vi "太阳能控制器界面.vi"() -> ()   [LabVIEW 2016, in "环境动力监测库.lvlib"]
uses:
  <vilib>/Utility/miscctls.llb/LVPointTypeDef.ctl
  <vilib>/Utility/config.llb/NI_LVConfig.lvlib
  <vilib>/ptbypt/NI_PtbyPt.lvlib
panel:
  in  "报警设置":bool
  in  "MPPT-24 串口":refnum<visa-resource-name> caption="MPPT-24"
  in  "MPPT-12 串口":refnum<visa-resource-name> caption="MPPT-12"
  out "充放电信息 2":T1 caption="充放电信息_KWH" {"总累计充电量" format="%.2f"; "当年累计充电量" format="%.2f"; "当月累计充电量" format="%.2f"; "当日累计充电量" format="%.2f"; "当年累计用电量" format="%.2f"; "当月累计用电量" format="%.2f"; "当日累计用电量" format="%.2f"}
  out "状态 2":string caption="状态"
  out "状态":string
  out "充放电信息":T1 caption="充放电信息_KWH" {"总累计充电量" format="%.2f"; "当年累计充电量" format="%.2f"; "当月累计充电量" format="%.2f"; "当日累计充电量" format="%.2f"; "当年累计用电量" format="%.2f"; "当月累计用电量" format="%.2f"; "当日累计用电量" format="%.2f"}
  out "通讯状态 3":bool
  out "通讯状态 2":bool
  out "控制器信息 2":cluster{"设备温度℃":dbl} caption="控制器信息"
  out "直流负载信息 2":cluster{"负载电压V":dbl, "负载电流A":dbl, "负载功率W":dbl} caption="直流负载信息"
  out "蓄电池信息 2":T2 caption="蓄电池信息"
  out "阵列信息 2":cluster{"阵列电压V":dbl, "阵列电流A":dbl, "发电功率W":dbl} caption="阵列信息"
  out "控制器信息":cluster{"设备温度℃":dbl}
  out "直流负载信息":cluster{"负载电压V":dbl, "负载电流A":dbl, "负载功率W":dbl}
  out "蓄电池信息":T2
  out "阵列信息":cluster{"阵列电压V":dbl, "阵列电流A":dbl, "发电功率W":dbl}
  # "MPPT-12"
  # "MPPT-24"
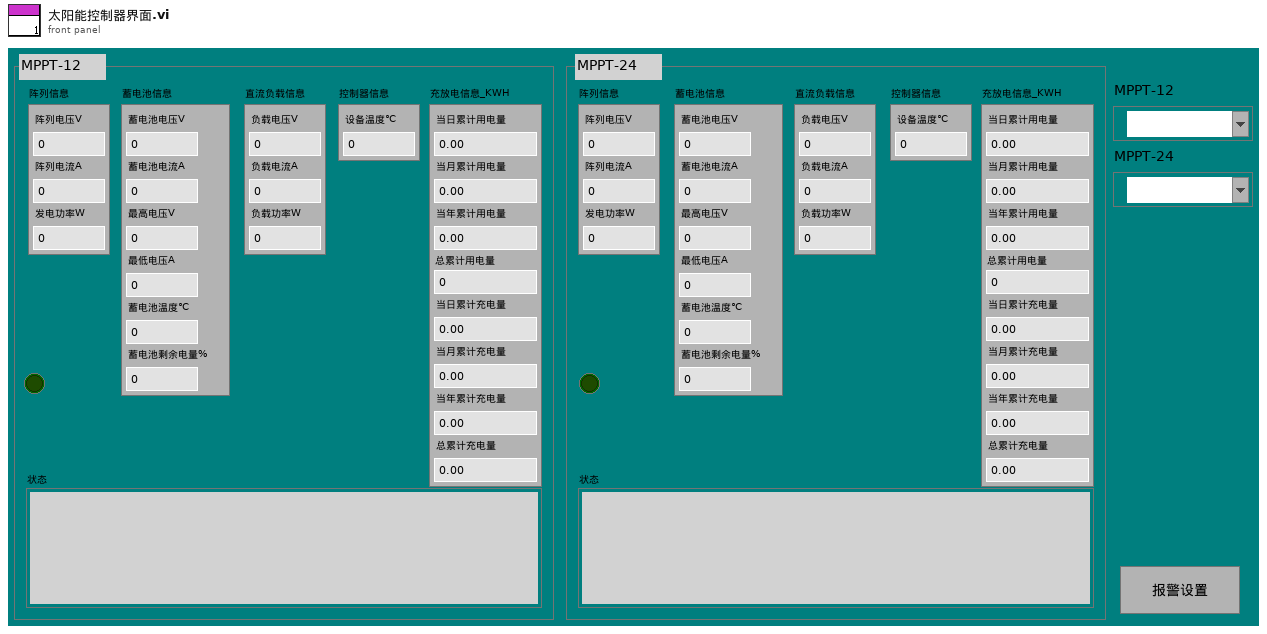
[diagram p1: front panel]
types:
  T1 = cluster{"当日累计用电量":sgl, "当月累计用电量":sgl, "当年累计用电量":sgl, "总累计用电量":sgl, "当日累计充电量":sgl, "当月累计充电量":sgl, "当年累计充电量":sgl, "总累计充电量":sgl}
  T2 = cluster{"蓄电池电压V":dbl, "蓄电池电流A":dbl, "最高电压V":dbl, "最低电压A":dbl, "蓄电池温度℃":dbl, "蓄电池剩余电量%":dbl}
  T3 = typedef "LVPointTypeDef.ctl" = cluster{"Horizontal":i16, "Vertical":i16}
  T4 = typedef "NI_LVConfig.lvlib/Config Data RefNum.ctl" = refnum<k1>
  T5 = enum8{"Enabled", "Disabled", "Disabled and Grayed Out"}
  T6 = cluster{"蓄电池状态":string, "阵列状态":string, "充电状态":string, "负载状态":string, "设备状态":string}
  T7 = cluster{"状态":cluster{"蓄电池状态":string, "阵列状态":string, "充电状态":string, "负载状态":string, "设备状态":string}, "充放电信息":cluster{"当日累计用电量":sgl, "当月累计用电量":sgl, "当年累计用电量":sgl, "总累计用电量":sgl, "当日累计充电量":sgl, "当月累计充电量":sgl, "当年累计充电量":sgl, "总累计充电量":sgl}, "控制器信息":cluster{"设备温度℃":dbl}, "蓄电池信息":cluster{"蓄电池电压V":dbl, "蓄电池电流A":dbl, "最高电压V":dbl, "最低电压A":dbl, "蓄电池温度℃":dbl, "蓄电池剩余电量%":dbl}, "阵列信息":cluster{"阵列电压V":dbl, "阵列电流A":dbl, "发电功率W":dbl}, "直流负载信息":cluster{"负载电压V":dbl, "负载电流A":dbl, "负载功率W":dbl}, "error out":errorcluster}
  T8 = cluster{"时间":timestamp, "阵列电压_V":dbl, "阵列电流_A":dbl, "发电功率_W":dbl, "蓄电池电压_V":dbl, "蓄电池电流_A":dbl, "最高电压_V":dbl, "最低电压_A":dbl, "蓄电池温度_℃":dbl, "蓄电池剩余电量_%":dbl, "负载电压_V":dbl, "负载电流_A":dbl, "负载功率_W":dbl, "设备温度_℃":dbl, "当日累计用电量_KWH":dbl, "当月累计用电量_KWH":dbl, "当年累计用电量_KWH":dbl, "总累计用电量_KWH":dbl, "当日累计充电量_KWH":dbl, "当月累计充电量_KWH":dbl, "当年累计充电量_KWH":dbl, "总累计充电量_KWH":dbl}
  T9 = typedef "LVDateTimeRec.ctl" = cluster{"秒数的小数部分":dbl, "秒":i32, "分":i32, "时":i32, "日":i32, "月":i32, "年":i32, "天数（周）":i32, "天数（年）":i32, "DST":i32}
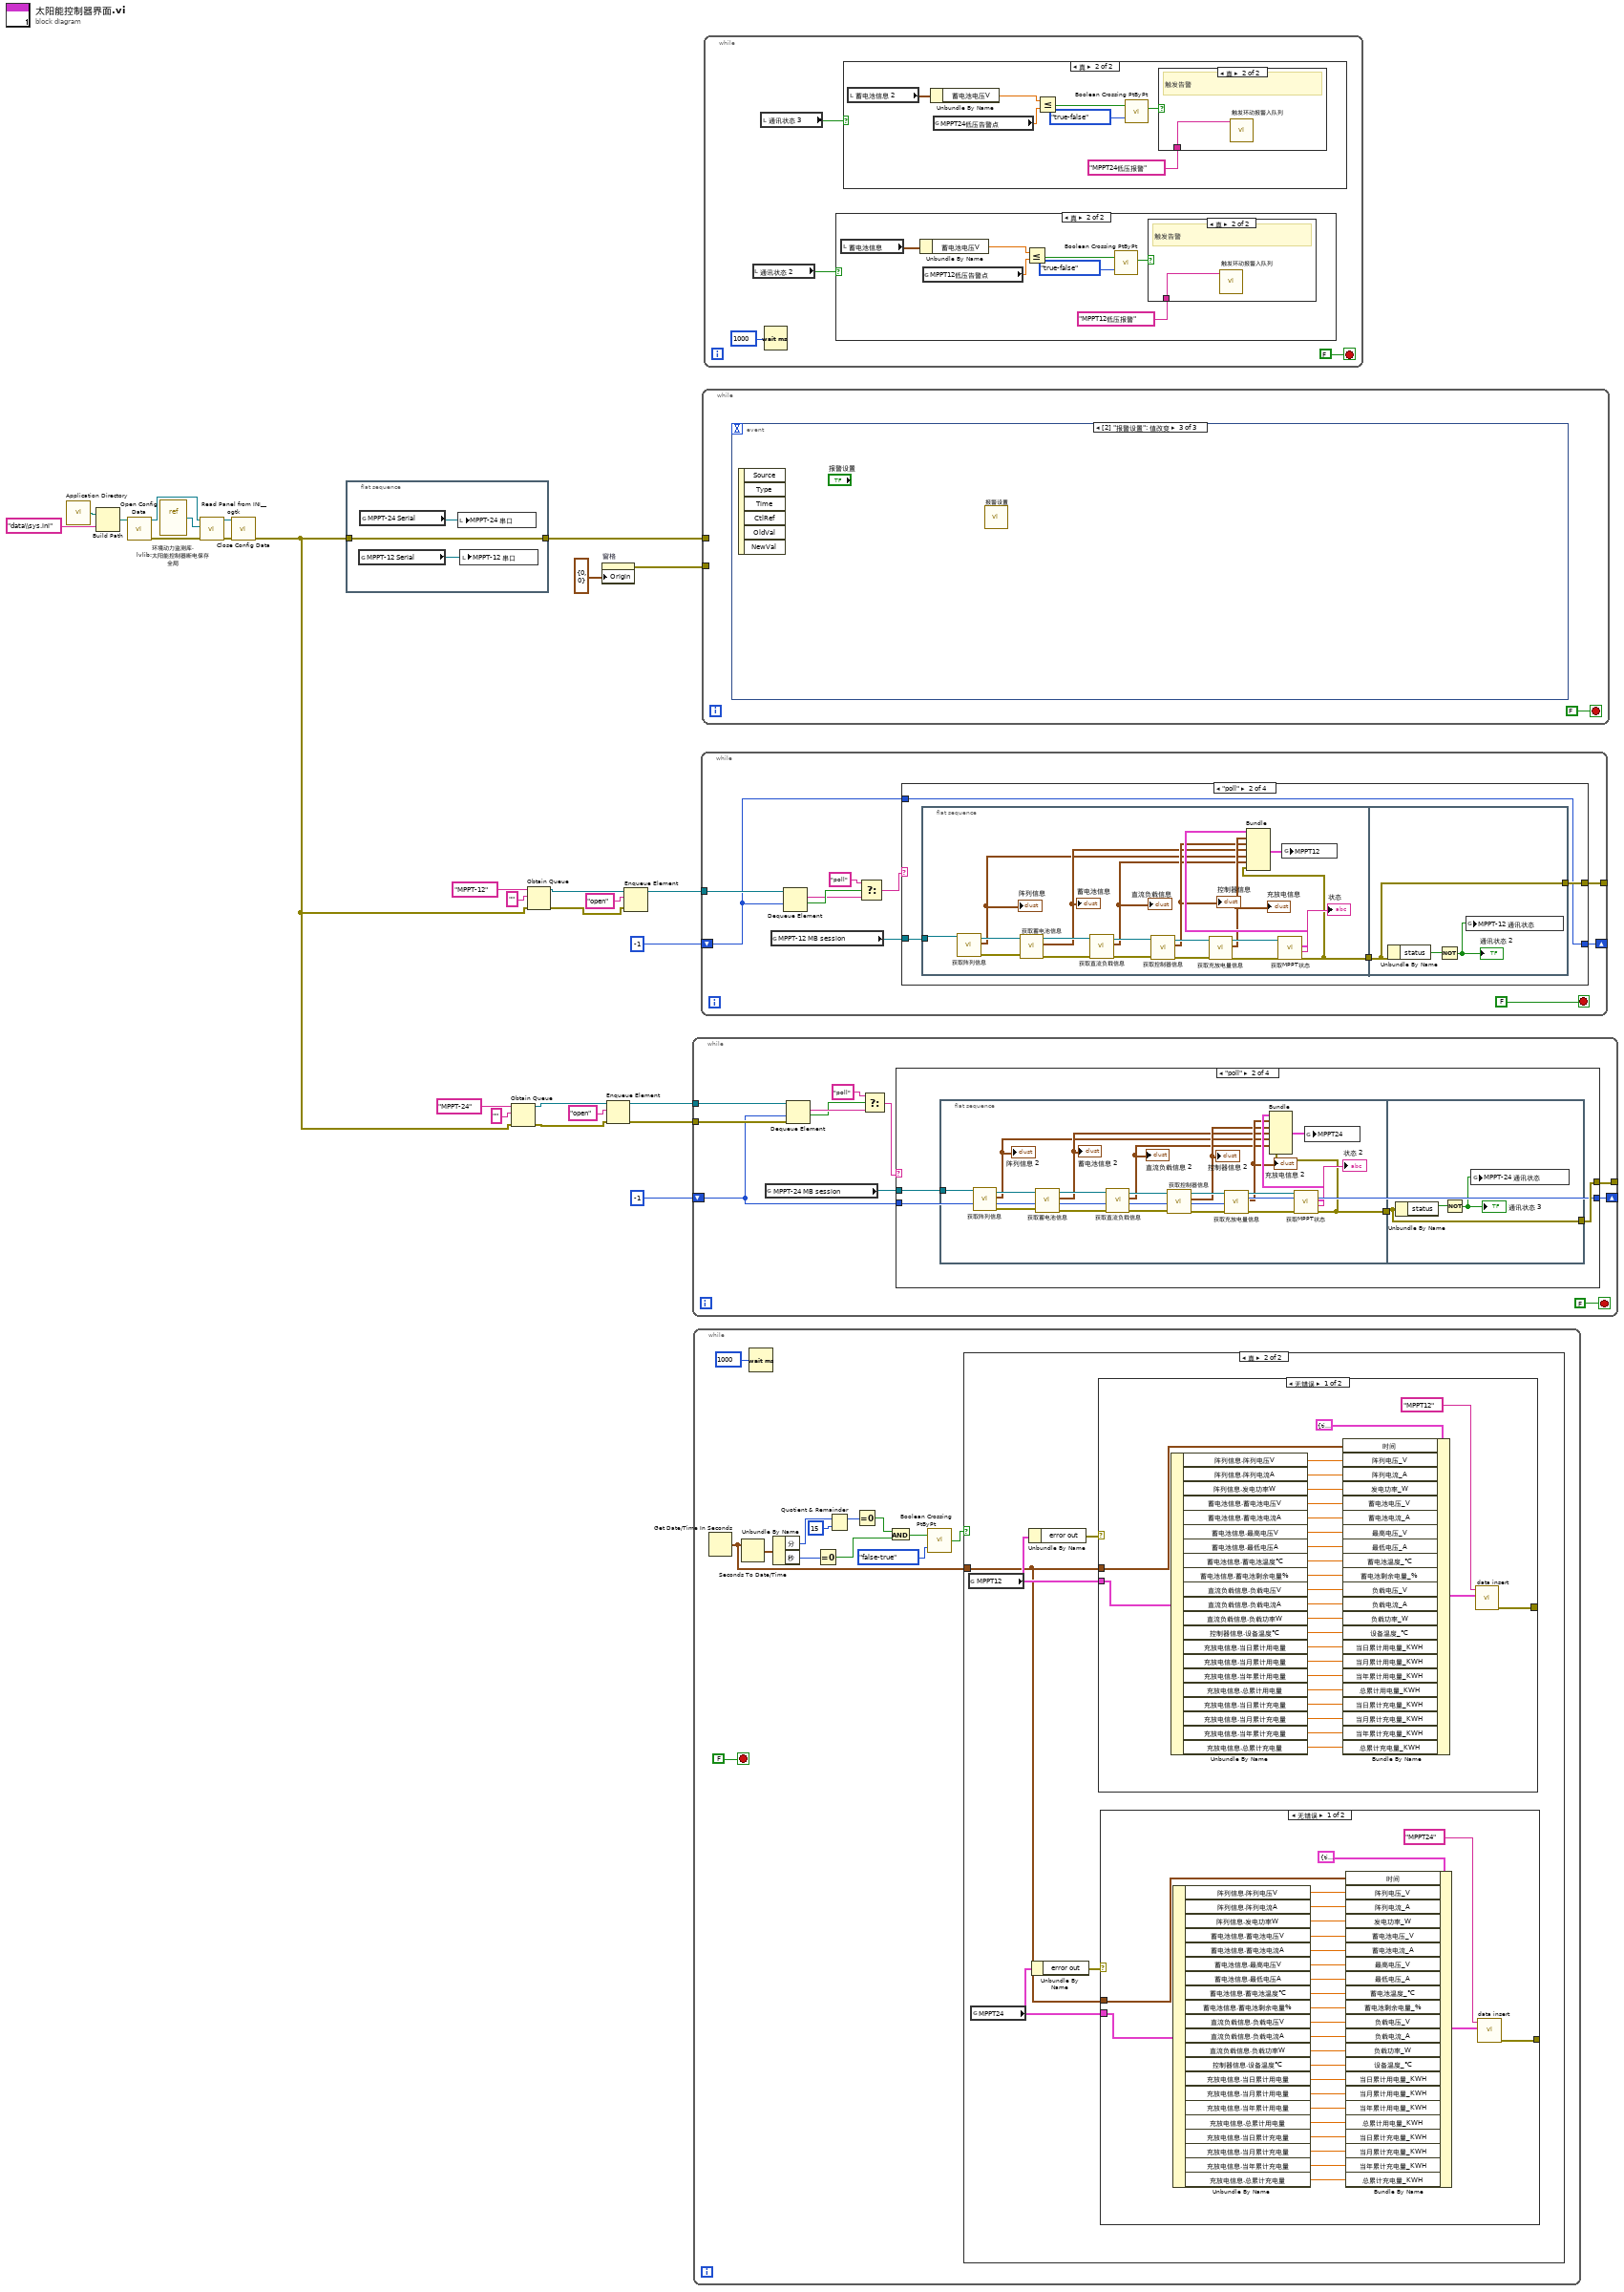
[diagram p0: block diagram]
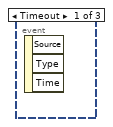
[diagram p9: hidden frame]
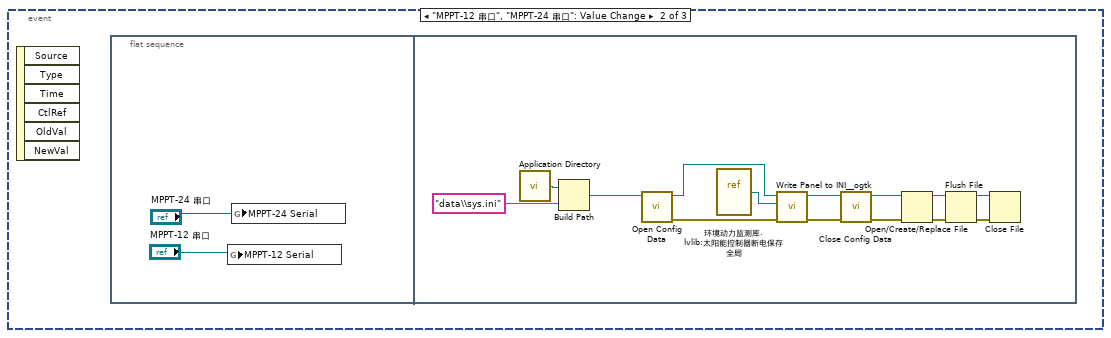
[diagram p10: hidden frame]
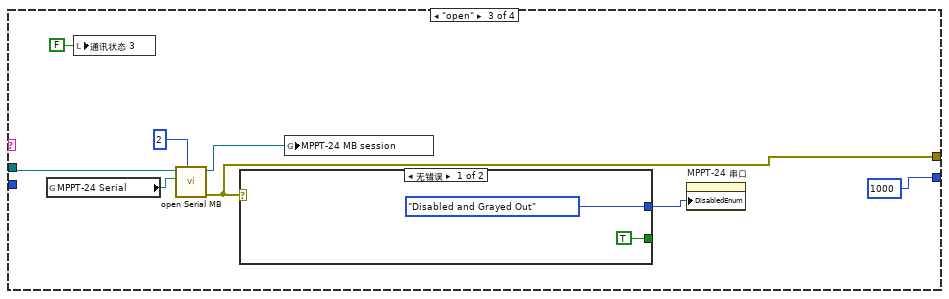
[diagram p12: hidden frame]
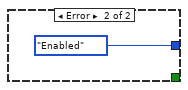
[diagram p13: hidden frame]
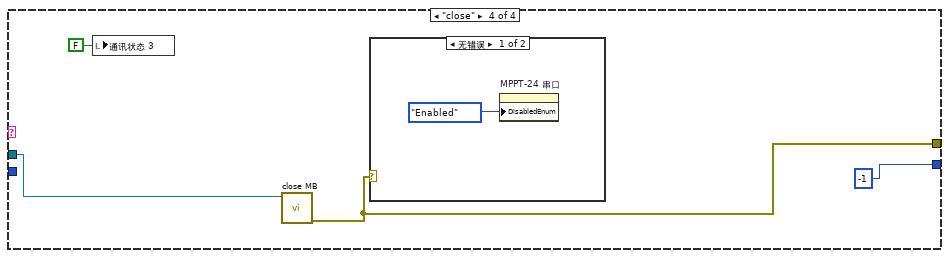
[diagram p14: hidden frame]
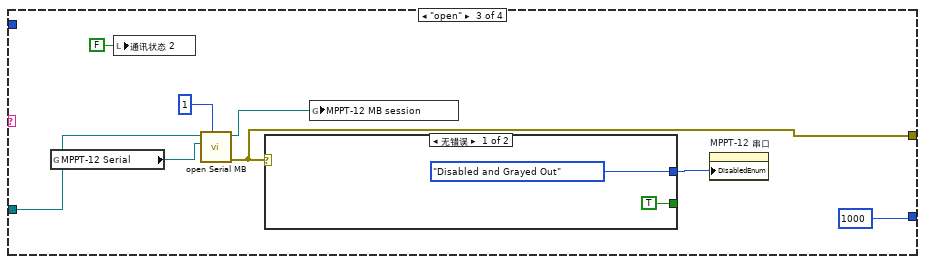
[diagram p17: hidden frame]
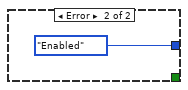
[diagram p18: hidden frame]
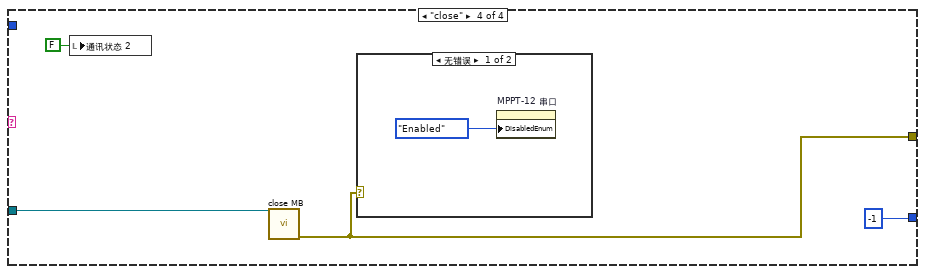
[diagram p19: hidden frame]
diagram:
  n1 = call <vilib>:"Application Directory.vi"() -> ("Application Directory"=w16:path)
  n2 = Build Path(base path=w16, name or relative path="data\\sys.ini" ("名称或相对路径")) -> (appended path=w18:path)
  n3 = call <vilib>:"Open Config Data.vi"("configuration file path"=w18) -> ("error out"=w22:errorcluster, "refnum"=w19:T4)  [unwired: 8 in, 1 out]
  n4 = vi-ref "环境动力监测库.lvlib:太阳能控制器断电保存全局.vi"() -> (w20:refnum<vi>)
  n5 = call <userlib>:"Read Panel from INI__ogtk.vi"("error in (no error)"=w22, "VI ref"=w20, "refnum"=w19) -> ("error out"=w15:errorcluster, "refnum out"=w21:T4)  [unwired: 7 in]
  n6 = call <vilib>:"Close Config Data.vi"("error in (no error)"=w15, "refnum"=w21) -> ("error out"=w2:errorcluster)  [unwired: 8 in, 1 out]
  n7 = flat-sequence {
    tunnel: w2 -> [w28]
    tunnel: [w28] -> w1
    frame #0 {
      n8 = global read "太阳能控制器断电保存全局.vi" "MPPT-12 Serial"() -> (w30:refnum<visa-resource-name>)
      n9 = global read "太阳能控制器断电保存全局.vi" "MPPT-24 Serial"() -> (w29:refnum<visa-resource-name>)
      n10 = local write "MPPT-24 串口"(w29) -> ()
      n11 = local write "MPPT-12 串口"(w30) -> ()
    }
  }
  n12 = Obtain Queue(name (unnamed)="MPPT-24" ("名称（未命名）"), element data type="", error in (no error)=w2) -> (queue out=w4:refnum<queue>, error out=w3:errorcluster)  [unwired: 2 in, 1 out]
  n13 = Obtain Queue(name (unnamed)="MPPT-12" ("名称（未命名）"), element data type="", error in (no error)=w2) -> (queue out=w6:refnum<queue>, error out=w5:errorcluster)  [unwired: 2 in, 1 out]
  n14 = property on="窗格" class="Pane"("Origin"=T3 {"Horizontal"=0, "Vertical"=0} ("原点")) -> (error out=w13:errorcluster)  [unwired: 2 in, 1 out]
  n15 = Enqueue Element(queue=w4, element="open" ("元素"), error in (no error)=w3) -> (queue out=w25:refnum<queue>, error out=w24:errorcluster)  [unwired: 1 in, 1 out]
  n16 = Enqueue Element(queue=w6, element="open" ("元素"), error in (no error)=w5) -> (queue out=w26:refnum<queue>)  [unwired: 1 in, 2 out]
  n17 = while {
    tunnel: w25 -> [w38]
    tunnel: w24 -> [w37]
    shift-right: [w33] -> _
    shift-left: -1 ("超时毫秒(-1)") -> [w31]
    tunnel: [w34] -> _
    stop <- FALSE stop-if-true
    n18 = global read "太阳能控制器全局.vi" "MPPT-24 MB session"() -> (w35:refnum<class "MB_Master.lvclass">)
    n19 = Dequeue Element(queue=w38, timeout in ms (-1)=w31, error in (no error)=w37) -> (element=w41:string, timed out?=w39:bool)  [unwired: 2 out]
    n20 = Select(t="poll" ("元素"), s=w39, f=w41) -> (s? t:f=w36:string)
    n21 = case shown="\"poll\"" w36 {
      tunnel: w35 -> [_ w46 w73 w83]
      tunnel: [_ w44 w72 w82] -> w34
      tunnel: [w42 w43 1000 ("超时毫秒(-1)") -1 ("超时毫秒(-1)")] -> w33
      tunnel: w31 -> [w42 w43 _ _]
      frame Default {
      }
      frame "poll" {
        n22 = flat-sequence {
          tunnel: w46 -> [w56]
          tunnel: [w47] -> w45
          tunnel: w45 -> [w67]
          tunnel: [w67] -> w44
          frame #0 {
            n23 = call "获取阵列信息.vi"("MB session in"=w56) -> ("error out"=w65:errorcluster, "阵列信息"=w49:cluster{"阵列电压V":dbl, "阵列电流A":dbl, "发电功率W":dbl}, "MB session out"=w66:refnum<class "MB_Master.lvclass">)  [unwired: 8 in]
            "阵列信息 2" <- w49
            n24 = call "获取蓄电池信息.vi"("error in (no error)"=w65, "MB session in"=w66) -> ("error out"=w63:errorcluster, "蓄电池信息"=w50:T2, "MB session out"=w64:refnum<class "MB_Master.lvclass">)  [unwired: 7 in]
            "蓄电池信息 2" <- w50
            n25 = call "获取直流负载信息.vi"("error in (no error)"=w63, "MB session in"=w64) -> ("error out"=w61:errorcluster, "直流负载信息"=w48:cluster{"负载电压V":dbl, "负载电流A":dbl, "负载功率W":dbl}, "MB session out"=w62:refnum<class "MB_Master.lvclass">)  [unwired: 7 in]
            "直流负载信息 2" <- w48
            n26 = call "获取控制器信息.vi"("error in (no error)"=w61, "MB session in"=w62) -> ("error out"=w59:errorcluster, "控制器信息"=w51:cluster{"设备温度℃":dbl}, "MB session out"=w60:refnum<class "MB_Master.lvclass">)  [unwired: 7 in]
            "控制器信息 2" <- w51
            n27 = call "获取充放电量信息.vi"("error in (no error)"=w59, "MB session in"=w60) -> ("error out"=w57:errorcluster, "充放电信息"=w52:T1, "MB session out"=w58:refnum<class "MB_Master.lvclass">)  [unwired: 7 in]
            "充放电信息 2" <- w52
            n28 = call "获取MPPT状态.vi"("error in (no error)"=w57, "MB session in"=w58) -> ("error out"=w47:errorcluster, "结果字符串"=→"状态 2":string, "状态"=w54:T6)  [unwired: 6 in, 1 out]
            n29 = Bundle("状态"=w54, "充放电信息"=w52, "控制器信息"=w51, "蓄电池信息"=w50, "阵列信息"=w49, "直流负载信息"=w48, "error out"=w47) -> (w53:T7)  [unwired: 1 in]
            n30 = global write "太阳能控制器全局.vi" "MPPT24"(w53) -> ()
          }
          frame #1 {
            n31 = Unbundle By Name(w67) -> ("status"=w69:bool)
            n32 = Not(x=w69) -> (.not. x?=w68:bool)
            "通讯状态 3" <- w68
            n33 = global write "太阳能控制器全局.vi" "MPPT-24 通讯状态"(w68) -> ()
          }
        }
      }
      frame "open" {
        n34 = global read "太阳能控制器断电保存全局.vi" "MPPT-24 Serial"() -> (w75:refnum<visa-resource-name>)
        n35 = local write "通讯状态 3"(FALSE ("通讯状态 3")) -> ()
        n36 = call "open Serial MB.vi"("Slave ID"=u8 2, "VISA Resource"=w75, "MB session in"=w73) -> ("error out"=w72:errorcluster, "MB session out"=w76:refnum<class "MB_Master.lvclass">)  [unwired: 7 in]
        n37 = case shown="无错误" w72 {
          tunnel: [T5."Disabled and Grayed Out" ("禁用") T5."Enabled" ("禁用")] -> w70
          tunnel: [TRUE _] -> _
          frame No Error {
          }
          frame Error {
          }
        }
        n38 = global write "太阳能控制器全局.vi" "MPPT-24 MB session"(w76) -> ()
        n39 = property on="MPPT-24 串口" class="VISAName"("DisabledEnum"=w70) -> ()  [unwired: 2 in, 2 out]
      }
      frame "close" {
        n40 = local write "通讯状态 3"(FALSE ("通讯状态 2")) -> ()
        n41 = call "close MB.vi"("MB session in"=w83) -> ("error out"=w82:errorcluster)  [unwired: 10 in]
        n42 = case shown="无错误" w82 {
          frame No Error {
            n43 = property on="MPPT-24 串口" class="VISAName"("DisabledEnum"=T5."Enabled" ("禁用")) -> ()  [unwired: 2 in, 2 out]
          }
          frame Error {
          }
        }
      }
    }
  }
  n44 = while {
    stop <- FALSE stop-if-true
    n45 = Get Date/Time In Seconds() -> (seconds since 1Jan1904=w86:timestamp)
    n46 = Seconds To Date/Time(time stamp (now)=w86) -> (date time rec=w96:T9)  [unwired: 1 in]
    n47 = Wait (ms)(milliseconds to wait=u32 1000 ("等待时间（毫秒）")) -> ()  [unwired: 1 out]
    n48 = Unbundle By Name(w96) -> ("分"=w95:i32, "秒"=w92:i32)
    n49 = Equal To 0?(x=w92) -> (x = 0?=w90:bool)
    n50 = Quotient & Remainder(x=w95, y=15) -> (x-y*floor(x/y)=w93:i32)  [unwired: 1 out]
    n51 = Equal To 0?(x=w93) -> (x = 0?=w91:bool)
    n52 = And(x=w91, y=w90) -> (x .and. y?=w89:bool)
    n53 = call <vilib>:"Boolean Crossing PtByPt.vi"("direction"=enum16{"either", "false-true", "true-false"}."false-true", "input"=w89) -> ("crossing"=w87:bool)  [unwired: 1 in]
    n54 = case shown="真" w87 {
      tunnel: w86 -> [_ w99]
      frame False {
      }
      frame True {
        n55 = global read "太阳能控制器全局.vi" "MPPT12"() -> (w102:T7)
        n56 = global read "太阳能控制器全局.vi" "MPPT24"() -> (w101:T7)
        n57 = Unbundle By Name(w102) -> ("error out"=w103:errorcluster)
        n58 = Unbundle By Name(w101) -> ("error out"=w100:errorcluster)
        n59 = case shown="无错误" w103 {
          tunnel: w102 -> [w135 _]
          tunnel: w99 -> [w134 _]
          tunnel: [w131 _] -> _
          frame No Error {
            n60 = Unbundle By Name(w135) -> ("阵列信息.阵列电压V"=w137:dbl, "阵列信息.阵列电流A"=w138:dbl, "阵列信息.发电功率W"=w139:dbl, "蓄电池信息.蓄电池电压V"=w140:dbl, "蓄电池信息.蓄电池电流A"=w141:dbl, "蓄电池信息.最高电压V"=w142:dbl, "蓄电池信息.最低电压A"=w143:dbl, "蓄电池信息.蓄电池温度℃"=w144:dbl, "蓄电池信息.蓄电池剩余电量%"=w145:dbl, "直流负载信息.负载电压V"=w146:dbl, "直流负载信息.负载电流A"=w147:dbl, "直流负载信息.负载功率W"=w148:dbl, "控制器信息.设备温度℃"=w149:dbl, "充放电信息.当日累计用电量"=w150:sgl, "充放电信息.当月累计用电量"=w151:sgl, "充放电信息.当年累计用电量"=w152:sgl, "充放电信息.总累计用电量"=w153:sgl, "充放电信息.当日累计充电量"=w154:sgl, "充放电信息.当月累计充电量"=w155:sgl, "充放电信息.当年累计充电量"=w156:sgl, "充放电信息.总累计充电量"=w157:sgl)
            n61 = Bundle By Name(cluster=T8 {"时间"=timestamp(0 s since 1904-01-01), "阵列电压_V"=0.0, "阵列电流_A"=0.0, "发电功率_W"=0.0, "蓄电池电压_V"=0.0, "蓄电池电流_A"=0.0, "最高电压_V"=0.0, "最低电压_A"=0.0, "蓄电池温度_℃"=0.0, "蓄电池剩余电量_%"=0.0, "负载电压_V"=0.0, "负载电流_A"=0.0, "负载功率_W"=0.0, "设备温度_℃"=0.0, "当日累计用电量_KWH"=0.0, "当月累计用电量_KWH"=0.0, "当年累计用电量_KWH"=0.0, "总累计用电量_KWH"=0.0, "当日累计充电量_KWH"=0.0, "当月累计充电量_KWH"=0.0, "当年累计充电量_KWH"=0.0, "总累计充电量_KWH"=0.0} ("data in"), "时间"=w134, "阵列电压_V"=w137, "阵列电流_A"=w138, "发电功率_W"=w139, "蓄电池电压_V"=w140, "蓄电池电流_A"=w141, "最高电压_V"=w142, "最低电压_A"=w143, "蓄电池温度_℃"=w144, "蓄电池剩余电量_%"=w145, "负载电压_V"=w146, "负载电流_A"=w147, "负载功率_W"=w148, "设备温度_℃"=w149, "当日累计用电量_KWH"=w150, "当月累计用电量_KWH"=w151, "当年累计用电量_KWH"=w152, "总累计用电量_KWH"=w153, "当日累计充电量_KWH"=w154, "当月累计充电量_KWH"=w155, "当年累计充电量_KWH"=w156, "总累计充电量_KWH"=w157) -> (w133:T8)
            n62 = call "data insert.vi"("data in"=w133, "table"="MPPT12") -> ("error out"=w131:errorcluster)  [unwired: 9 in]
          }
          frame Error {
          }
        }
        n63 = case shown="无错误" w100 {
          tunnel: w101 -> [w108 _]
          tunnel: w99 -> [w107 _]
          tunnel: [w104 _] -> _
          frame No Error {
            n64 = Unbundle By Name(w108) -> ("阵列信息.阵列电压V"=w110:dbl, "阵列信息.阵列电流A"=w111:dbl, "阵列信息.发电功率W"=w112:dbl, "蓄电池信息.蓄电池电压V"=w113:dbl, "蓄电池信息.蓄电池电流A"=w114:dbl, "蓄电池信息.最高电压V"=w115:dbl, "蓄电池信息.最低电压A"=w116:dbl, "蓄电池信息.蓄电池温度℃"=w117:dbl, "蓄电池信息.蓄电池剩余电量%"=w118:dbl, "直流负载信息.负载电压V"=w119:dbl, "直流负载信息.负载电流A"=w120:dbl, "直流负载信息.负载功率W"=w121:dbl, "控制器信息.设备温度℃"=w122:dbl, "充放电信息.当日累计用电量"=w123:sgl, "充放电信息.当月累计用电量"=w124:sgl, "充放电信息.当年累计用电量"=w125:sgl, "充放电信息.总累计用电量"=w126:sgl, "充放电信息.当日累计充电量"=w127:sgl, "充放电信息.当月累计充电量"=w128:sgl, "充放电信息.当年累计充电量"=w129:sgl, "充放电信息.总累计充电量"=w130:sgl)
            n65 = Bundle By Name(cluster=T8 {"时间"=timestamp(0 s since 1904-01-01), "阵列电压_V"=0.0, "阵列电流_A"=0.0, "发电功率_W"=0.0, "蓄电池电压_V"=0.0, "蓄电池电流_A"=0.0, "最高电压_V"=0.0, "最低电压_A"=0.0, "蓄电池温度_℃"=0.0, "蓄电池剩余电量_%"=0.0, "负载电压_V"=0.0, "负载电流_A"=0.0, "负载功率_W"=0.0, "设备温度_℃"=0.0, "当日累计用电量_KWH"=0.0, "当月累计用电量_KWH"=0.0, "当年累计用电量_KWH"=0.0, "总累计用电量_KWH"=0.0, "当日累计充电量_KWH"=0.0, "当月累计充电量_KWH"=0.0, "当年累计充电量_KWH"=0.0, "总累计充电量_KWH"=0.0} ("data in"), "时间"=w107, "阵列电压_V"=w110, "阵列电流_A"=w111, "发电功率_W"=w112, "蓄电池电压_V"=w113, "蓄电池电流_A"=w114, "最高电压_V"=w115, "最低电压_A"=w116, "蓄电池温度_℃"=w117, "蓄电池剩余电量_%"=w118, "负载电压_V"=w119, "负载电流_A"=w120, "负载功率_W"=w121, "设备温度_℃"=w122, "当日累计用电量_KWH"=w123, "当月累计用电量_KWH"=w124, "当年累计用电量_KWH"=w125, "总累计用电量_KWH"=w126, "当日累计充电量_KWH"=w127, "当月累计充电量_KWH"=w128, "当年累计充电量_KWH"=w129, "总累计充电量_KWH"=w130) -> (w106:T8)
            n66 = call "data insert.vi"("data in"=w106, "table"="MPPT24") -> ("error out"=w104:errorcluster)  [unwired: 9 in]
          }
          frame Error {
          }
        }
      }
    }
  }
  n67 = while {
    shift-right: [w158] -> _
    shift-left: -1 ("超时毫秒(-1)") -> [w159]
    tunnel: w26 -> [w164]
    tunnel: [w160] -> _
    stop <- FALSE stop-if-true
    n68 = global read "太阳能控制器全局.vi" "MPPT-12 MB session"() -> (w161:refnum<class "MB_Master.lvclass">)
    n69 = Dequeue Element(queue=w164, timeout in ms (-1)=w159) -> (element=w165:string, timed out?=w167:bool)  [unwired: 1 in, 2 out]
    n70 = Select(t="poll" ("元素"), s=w167, f=w165) -> (s? t:f=w162:string)
    n71 = case shown="\"poll\"" w162 {
      tunnel: w161 -> [_ w172 w202 w209]
      tunnel: [_ w170 w198 w207] -> w160
      tunnel: w159 -> [w168 w169 _ _]
      tunnel: [w168 w169 1000 ("超时毫秒(-1)") -1 ("超时毫秒(-1)")] -> w158
      frame Default {
      }
      frame "poll" {
        n72 = flat-sequence {
          tunnel: w172 -> [w192]
          tunnel: [w174] -> w171
          tunnel: w171 -> [w193]
          tunnel: [w193] -> w170
          frame #0 {
            n73 = call "获取阵列信息.vi"("MB session in"=w192) -> ("error out"=w190:errorcluster, "阵列信息"=w176:cluster{"阵列电压V":dbl, "阵列电流A":dbl, "发电功率W":dbl}, "MB session out"=w191:refnum<class "MB_Master.lvclass">)  [unwired: 8 in]
            "阵列信息" <- w176
            n74 = call "获取蓄电池信息.vi"("error in (no error)"=w190, "MB session in"=w191) -> ("error out"=w188:errorcluster, "蓄电池信息"=w177:T2, "MB session out"=w189:refnum<class "MB_Master.lvclass">)  [unwired: 7 in]
            "蓄电池信息" <- w177
            n75 = call "获取直流负载信息.vi"("error in (no error)"=w188, "MB session in"=w189) -> ("error out"=w186:errorcluster, "直流负载信息"=w175:cluster{"负载电压V":dbl, "负载电流A":dbl, "负载功率W":dbl}, "MB session out"=w187:refnum<class "MB_Master.lvclass">)  [unwired: 7 in]
            "直流负载信息" <- w175
            n76 = call "获取控制器信息.vi"("error in (no error)"=w186, "MB session in"=w187) -> ("error out"=w184:errorcluster, "控制器信息"=w178:cluster{"设备温度℃":dbl}, "MB session out"=w185:refnum<class "MB_Master.lvclass">)  [unwired: 7 in]
            "控制器信息" <- w178
            n77 = call "获取充放电量信息.vi"("error in (no error)"=w184, "MB session in"=w185) -> ("error out"=w182:errorcluster, "充放电信息"=w179:T1, "MB session out"=w183:refnum<class "MB_Master.lvclass">)  [unwired: 7 in]
            "充放电信息" <- w179
            n78 = call "获取MPPT状态.vi"("error in (no error)"=w182, "MB session in"=w183) -> ("error out"=w174:errorcluster, "结果字符串"=→"状态":string, "状态"=w180:T6)  [unwired: 6 in, 1 out]
            n79 = Bundle("状态"=w180, "充放电信息"=w179, "控制器信息"=w178, "蓄电池信息"=w177, "阵列信息"=w176, "直流负载信息"=w175, "error out"=w174) -> (w173:T7)  [unwired: 1 in]
            n80 = global write "太阳能控制器全局.vi" "MPPT12"(w173) -> ()
          }
          frame #1 {
            n81 = Unbundle By Name(w193) -> ("status"=w195:bool)
            n82 = Not(x=w195) -> (.not. x?=w194:bool)
            "通讯状态 2" <- w194
            n83 = global write "太阳能控制器全局.vi" "MPPT-12 通讯状态"(w194) -> ()
          }
        }
      }
      frame "open" {
        n84 = global read "太阳能控制器断电保存全局.vi" "MPPT-12 Serial"() -> (w196:refnum<visa-resource-name>)
        n85 = local write "通讯状态 2"(FALSE ("通讯状态 2")) -> ()
        n86 = call "open Serial MB.vi"("Slave ID"=u8 1, "VISA Resource"=w196, "MB session in"=w202) -> ("error out"=w198:errorcluster, "MB session out"=w200:refnum<class "MB_Master.lvclass">)  [unwired: 7 in]
        n87 = case shown="无错误" w198 {
          tunnel: [T5."Disabled and Grayed Out" ("禁用") T5."Enabled" ("禁用")] -> w199
          tunnel: [TRUE _] -> _
          frame No Error {
          }
          frame Error {
          }
        }
        n88 = global write "太阳能控制器全局.vi" "MPPT-12 MB session"(w200) -> ()
        n89 = property on="MPPT-12 串口" class="VISAName"("DisabledEnum"=w199) -> ()  [unwired: 2 in, 2 out]
      }
      frame "close" {
        n90 = local write "通讯状态 2"(FALSE ("通讯状态 2")) -> ()
        n91 = call "close MB.vi"("MB session in"=w209) -> ("error out"=w207:errorcluster)  [unwired: 10 in]
        n92 = case shown="无错误" w207 {
          frame No Error {
            n93 = property on="MPPT-12 串口" class="VISAName"("DisabledEnum"=T5."Enabled" ("禁用")) -> ()  [unwired: 2 in, 2 out]
          }
          frame Error {
          }
        }
      }
    }
  }
  n94 = while {
    tunnel: w13 -> [_]
    tunnel: w1 -> [_]
    stop <- FALSE stop-if-true
    n95 = event shown="[2] \"报警设置\": 值改变" {
      selector: _ -> [_ _ _]
      dyn-events: _ -> [_ _ _]
      timeout: _ -> [_ _ _]
      event Timeout {
        n96 = event-data() -> ()  [unwired: 1 in, 3 out]
      }
      event "MPPT-12 串口", "MPPT-24 串口": Value Change {
        n97 = event-data() -> ()  [unwired: 1 in, 6 out]
        n98 = flat-sequence {
          frame #0 {
            n99 = global write "太阳能控制器断电保存全局.vi" "MPPT-12 Serial"("MPPT-12 串口") -> ()
            n100 = global write "太阳能控制器断电保存全局.vi" "MPPT-24 Serial"("MPPT-24 串口") -> ()
          }
          frame #1 {
            n101 = call <vilib>:"Application Directory.vi"() -> ("Application Directory"=w228:path)
            n102 = Build Path(base path=w228, name or relative path="data\\sys.ini" ("名称或相对路径")) -> (appended path=w226:path)
            n103 = call <vilib>:"Open Config Data.vi"("configuration file path"=w226) -> ("error out"=w222:errorcluster, "refnum"=w225:T4)  [unwired: 8 in, 1 out]
            n104 = vi-ref "环境动力监测库.lvlib:太阳能控制器断电保存全局.vi"() -> (w224:refnum<vi>)
            n105 = call <userlib>:"Write Panel to INI__ogtk.vi"("error in (no error)"=w222, "VI ref"=w224, "refnum"=w225) -> ("error out"=w221:errorcluster, "refnum out"=w223:T4)  [unwired: 7 in]
            n106 = call <vilib>:"Close Config Data.vi"("error in (no error)"=w221, "refnum"=w223) -> ("error out"=w216:errorcluster, "file path"=w215:path)  [unwired: 8 in]
            n107 = Open/Create/Replace File(file path (use dialog)=w215, error in=w216) -> (refnum out=w219:refnum<file>, error out=w220:errorcluster)  [unwired: 4 in, 1 out]
            n108 = Flush File(refnum=w219, error in=w220) -> (refnum out=w218:refnum<file>, error out=w217:errorcluster)
            n109 = Close File(refnum=w218, error in=w217) -> ()  [unwired: 2 out]
          }
        }
      }
      event "报警设置": Value Change {
        n110 = event-data() -> ()  [unwired: 1 in, 6 out]
        n111 = call "报警设置.vi"() -> ()  [unwired: 12 in]
      }
    }
  }
  n112 = while {
    stop <- FALSE stop-if-true
    n113 = local read "通讯状态 2"() -> (w230:bool)
    n114 = local read "通讯状态 3"() -> (w229:bool)
    n115 = Wait (ms)(milliseconds to wait=u32 1000 ("等待时间（毫秒）")) -> ()  [unwired: 1 out]
    n116 = case shown="真" w230 {
      frame False {
      }
      frame True {
        n117 = local read "蓄电池信息"() -> (w247:T2)
        n118 = Unbundle By Name(w247) -> ("蓄电池电压V"=w244:dbl)
        n119 = global read "太阳能控制器断电保存全局.vi" "MPPT12低压告警点"() -> (w243:dbl)
        n120 = Less Or Equal?(x=w244, y=w243) -> (x <= y?=w242:bool)
        n121 = call <vilib>:"Boolean Crossing PtByPt.vi"("direction"=enum16{"either", "false-true", "true-false"}."true-false", "input"=w242) -> ("crossing"=w245:bool)  [unwired: 1 in]
        n122 = case shown="真" w245 {
          tunnel: "MPPT12低压报警" ("设备") -> [_ w248]
          frame False {
          }
          frame True {
            # "触发告警"
            n123 = call "触发环动报警入队列.vi"("报警内容"=w248) -> ()  [unwired: 11 in]
          }
        }
      }
    }
    n124 = case shown="真" w229 {
      frame False {
      }
      frame True {
        n125 = local read "蓄电池信息 2"() -> (w239:T2)
        n126 = Unbundle By Name(w239) -> ("蓄电池电压V"=w236:dbl)
        n127 = global read "太阳能控制器断电保存全局.vi" "MPPT24低压告警点"() -> (w235:dbl)
        n128 = Less Or Equal?(x=w236, y=w235) -> (x <= y?=w234:bool)
        n129 = call <vilib>:"Boolean Crossing PtByPt.vi"("direction"=enum16{"either", "false-true", "true-false"}."true-false", "input"=w234) -> ("crossing"=w237:bool)  [unwired: 1 in]
        n130 = case shown="真" w237 {
          tunnel: "MPPT24低压报警" ("设备") -> [_ w240]
          frame False {
          }
          frame True {
            # "触发告警"
            n131 = call "触发环动报警入队列.vi"("报警内容"=w240) -> ()  [unwired: 11 in]
          }
        }
      }
    }
  }
